vi "UTILITY Check Robocopy Run.vi"(8 "error in (no error)":errorcluster, 10 "Refresh Programs Named":string, 11 "Robocopy Location Command":string="C:\\Newfi Exe\\Robocopy Update.bat") -> (0 "error out":errorcluster)   [LabVIEW 2014]
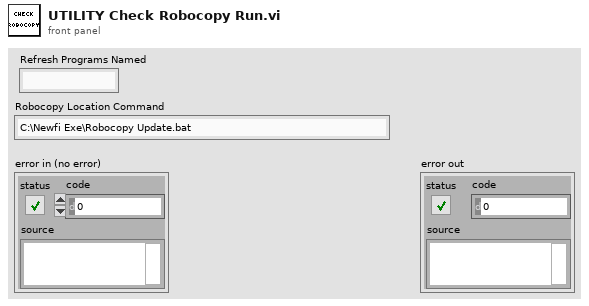
[diagram p1: front panel]
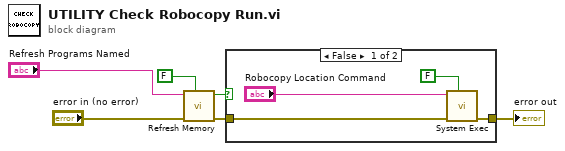
[diagram p0: block diagram]
diagram:
  n1 = call "Refresh Memory.vi"("Refresh?"=FALSE, "Error In"="error in (no error)", "Refresh Programs Named"="Refresh Programs Named") -> ("Error Out"=w4:errorcluster, "Do not Robocopy"=w2:bool)  [unwired: 7 in]
  n2 = case shown="False" w2 {
    tunnel: [w8 w11] -> w6
    tunnel: w4 -> [w7 w11]
    frame False {
      n3 = call <vilib>:"System Exec.vi"("wait until completion? (T)"=FALSE, "error in (no error)"=w7, "command line"="Robocopy Location Command") -> ("error out"=w8:errorcluster)  [unwired: 5 in, 3 out]
    }
    frame True {
    }
  }
  "error out" <- w6
